vi "Adquisición de velocidad.vi"() -> ()   [LabVIEW 2019]
uses:
  <vilib>/NI/Modbus Library/API/Wrapper/Create Serial Master.vi
  <vilib>/Waveform/WDTOps.llb/WDT Append Waveforms DBL.vi
  <vilib>/NI/Modbus Library/API/Master/Modbus Master.lvclass
  <vilib>/NI/Modbus Library/API/Wrapper/API Main.lvlib
panel:
  out "Frecuencia VFD":dbl
  in  "Reset Frecuencia":bool
  in  "Frecuencia automatica":bool
  out "Velocidad Medida r.p.m.":dbl(knob) scale=0.0..2100.0
  in  "VFD":bool
  in  "Frequency":dbl(knob) step=1.0 scale=0.0..75.0
  in  "stop 2":bool
  in  "Baud rate":u32=9600
  in  "Puerto":refnum<visa-resource-name>
  out "Velocidad medida (rpm)":dbl
  out "Frecuencia":dbl
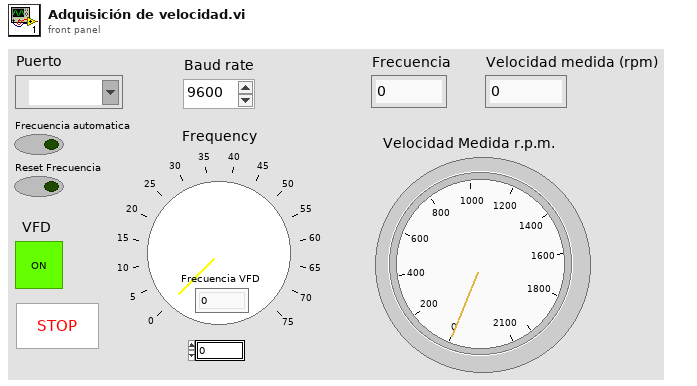
[diagram p1: front panel]
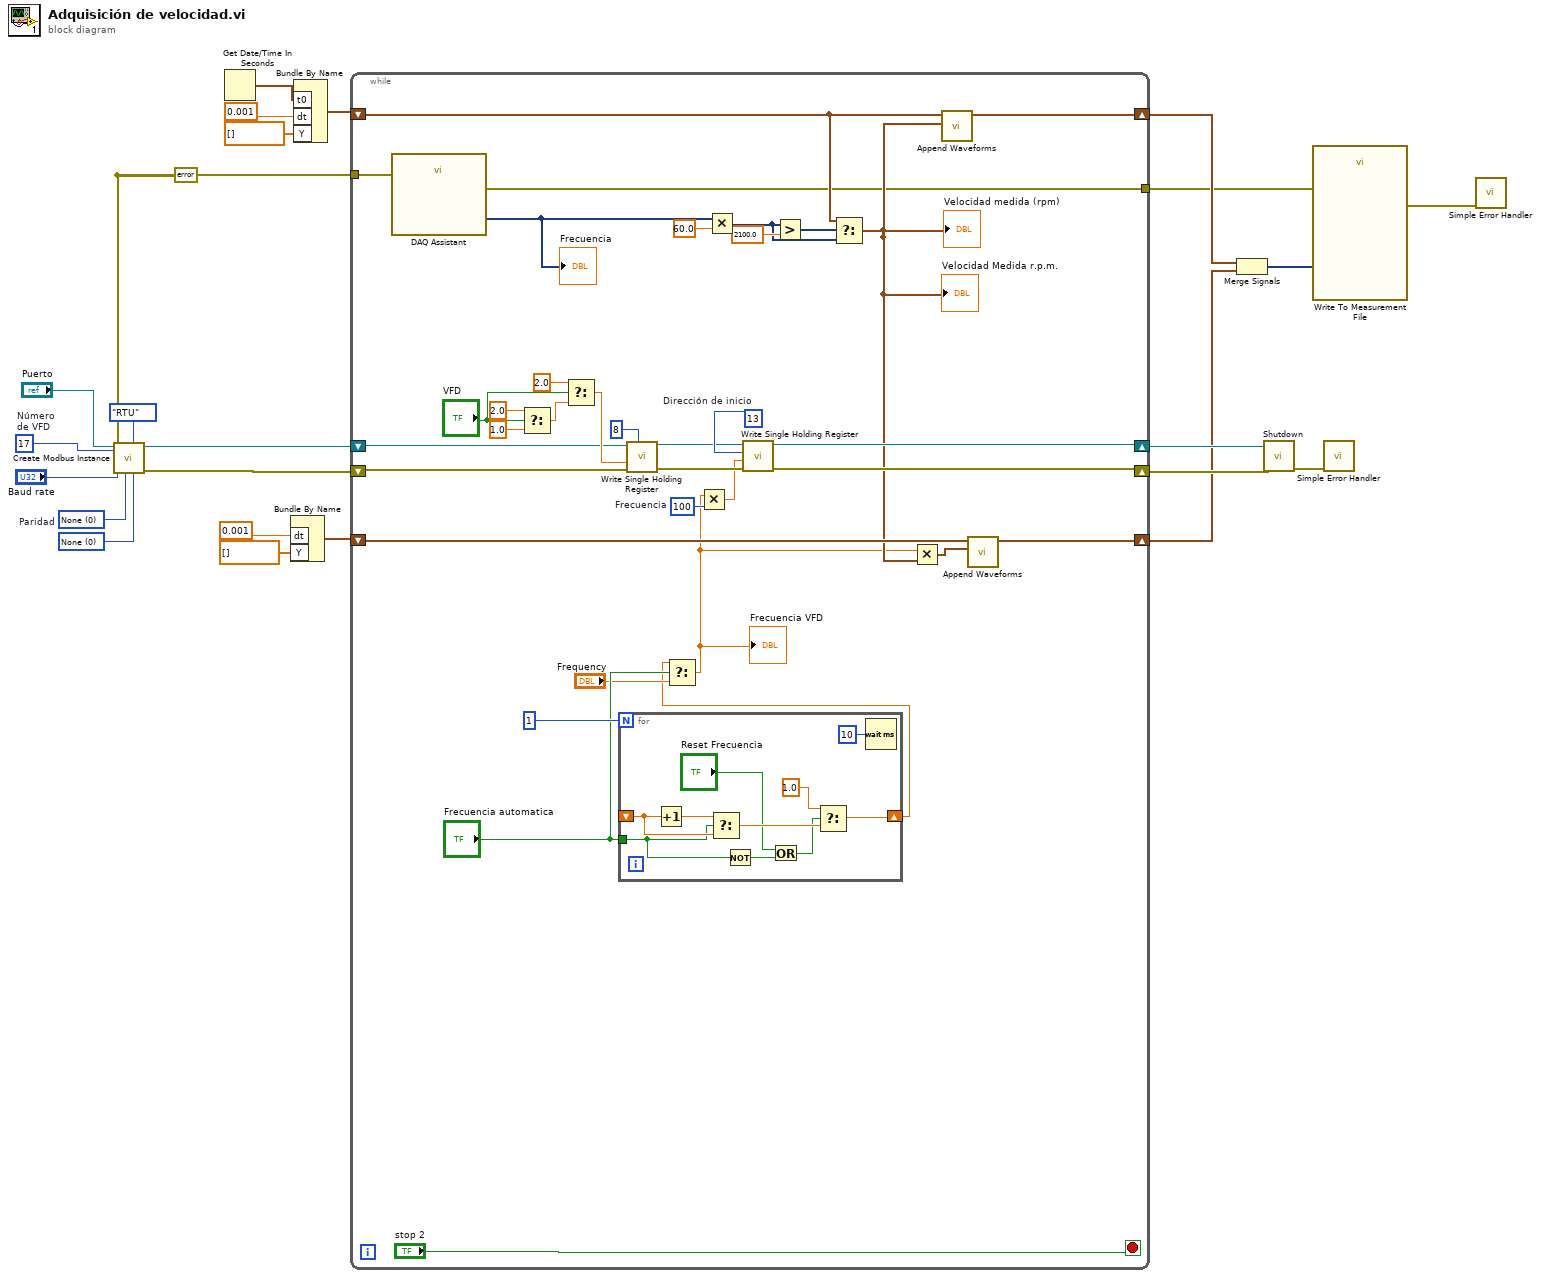
[diagram p0: block diagram]
diagram:
  w20 = u16 0 items=["None", "Odd", "Even", "Mark", "Space"]  # Paridad
  w21 = u16 0 items=["None", "XON/XOFF", "RTS/CTS", "XON/XOFF & RTS/CTS", "DTR/DSR", "XON/XOFF & DTR/DSR"] ("flow control (none)")
  w18 = errorcluster {"status"=FALSE, "code"=0, "source"=""} ("error in")
  w19 = u8 17  # Número de VFD
  n1 = call-poly <vilib>:"Create Modbus Instance.vi"("flow control (none)"=w21, "serial type"=enum16{"RTU", "ASCII"}."RTU", "parity (even)"=w20, "unit ID"=w19, "error in"=w18, "baud rate"="Baud rate", "VISA resource name"="Puerto") -> ("error out"=w16:errorcluster, "serial master instance"=w17:refnum<class "Modbus Master.lvclass">)  [unwired: 3 in]
  n2 = Get Date/Time In Seconds() -> (seconds since 1Jan1904=w10:timestamp)
  n3 = Bundle By Name("dt"=0.001, "Y"=dbl[] []) -> (w6:waveform(dbl))  [unwired: 1 in]
  n4 = Bundle By Name("t0"=w10, "dt"=0.001, "Y"=dbl[] []) -> (w9:waveform(dbl))  [unwired: 1 in]
  n5 = while {
    tunnel: w18 -> [w29]
    tunnel: [w27] -> w2
    shift-right: [w40] -> w5
    shift-left: w9 -> [w39]
    shift-right: [w42] -> w13
    shift-left: w17 -> [w44]
    shift-right: [w41] -> w14
    shift-left: w16 -> [w43]
    shift-right: [w37] -> w4
    shift-left: w6 -> [w38]
    stop <- "stop 2" stop-if-true
    w49 = u16 100  # Frecuencia
    w54 = u16 13  # Dirección de inicio
    n6 = call "DAQ Assistant"("error in"=w29) -> ("data"=w28:dynamicdata, "error out"=w27:errorcluster)  [unwired: 16 in, 1 out]
    "Frecuencia" <- w28
    n7 = Select(t=2.0, s="VFD", f=1.0) -> (s? t:f=w46:dbl)
    n8 = Select(t=2.0, s="VFD", f=w46) -> (s? t:f=w47:dbl)
    n9 = for {
      N: 1 -> [_]
      shift-right: [w66] -> w31
      shift-left: _ -> [w65]
      tunnel: "Frecuencia automatica" -> [w60]
      n10 = Increment(x=w65) -> (x+1=w68:dbl)
      n11 = Select(t=w68, s=w60, f=w65) -> (s? t:f=w67:dbl)
      n12 = Not(x=w60) -> (.not. x?=w61:bool)
      n13 = Or(x="Reset Frecuencia", y=w61) -> (x .or. y?=w63:bool)
      n14 = Select(t=1.0, s=w63, f=w67) -> (s? t:f=w66:dbl)
      n15 = Wait (ms)(milliseconds to wait=u32 10) -> ()  [unwired: 1 out]
    }
    n16 = call-dynamic "Write Single Holding Register.vi"("error in"=w43, "register to write"=w47, "address"=u16 8 ("Start"), "Modbus master in"=w44) -> ("error out"=w52:errorcluster, "Modbus master out"=w53:refnum<class "Modbus Master.lvclass">)  [unwired: 6 in]
    n17 = Select(t=w31, s="Frecuencia automatica", f="Frequency") -> (s? t:f=w30:dbl)
    "Frecuencia VFD" <- w30
    n18 = Multiply(x=w30, y=w49) -> (x*y=w48:dbl)
    n19 = Multiply(x=w28, y=60.0) -> (x*y=w56:dynamicdata)
    n20 = call-dynamic "Write Single Holding Register.vi"("error in"=w52, "register to write"=w48, "address"=w54, "Modbus master in"=w53) -> ("error out"=w41:errorcluster, "Modbus master out"=w42:refnum<class "Modbus Master.lvclass">)  [unwired: 6 in]
    n21 = Greater?(x=w56, y=2100.0) -> (0:w57:dynamicdata)
    n22 = Select(t=w39, s=w57, f=w56) -> (s? t:f=w36:waveform(dbl))
    "Velocidad medida (rpm)" <- w36
    "Velocidad Medida r.p.m." <- w36
    n23 = Multiply(x=w30, y=w36) -> (x*y=w35:waveform(dbl))
    n24 = call-poly <vilib>:"Append Waveforms.vi"("waveform B"=w36, "waveform A"=w39) -> ("waveform out"=w40:waveform(dbl))  [unwired: 8 in, 1 out]
    n25 = call-poly <vilib>:"Append Waveforms.vi"("waveform B"=w35, "waveform A"=w38) -> ("waveform out"=w37:waveform(dbl))  [unwired: 8 in, 1 out]
  }
  n26 = Merge Signals(w5, w4) -> (w1:dynamicdata)
  n27 = call-dynamic "Shutdown.vi"("error in"=w14, "Modbus master in"=w13) -> ("error out"=w15:errorcluster)  [unwired: 9 in]
  n28 = call "Write To Measurement File"("Signals"=w1, "error in (no error)"=w2) -> ("error out"=w3:errorcluster)  [unwired: 15 in, 2 out]
  n29 = call <vilib>:"Simple Error Handler.vi"("error in (no error)"=w15) -> ()  [unwired: 4 in, 5 out]
  n30 = call <vilib>:"Simple Error Handler.vi"("error in (no error)"=w3) -> ()  [unwired: 4 in, 5 out]
